vi "Create Token Request.vi"(4 "Code":string, 6 "State":string, 10 "Client":refnum<class "Client.lvclass">, 11 "Request in":refnum<class "Request.lvclass">) -> (1 "error out":errorcluster, 2 "POST Buffer":string, 3 "Request URL":string)   [LabVIEW 2020, in "OAuth2.lvlib" / "Request.lvclass"]
doc: "Internal VI for creating the URL and POST request body for performing a token request. This VI is only needed if implementing customized authorization flow functionality."
uses:
  Request.lvclass
  lv-http-util/HTTP Utils/HTTP Utils.lvlib
  Client/Client.lvclass
  lv-stream/stream/URI/URI.lvclass
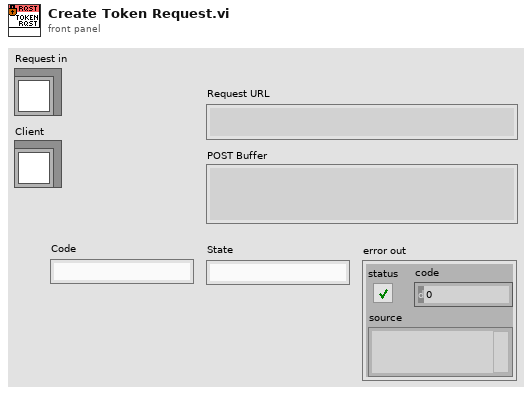
[diagram p1: front panel]
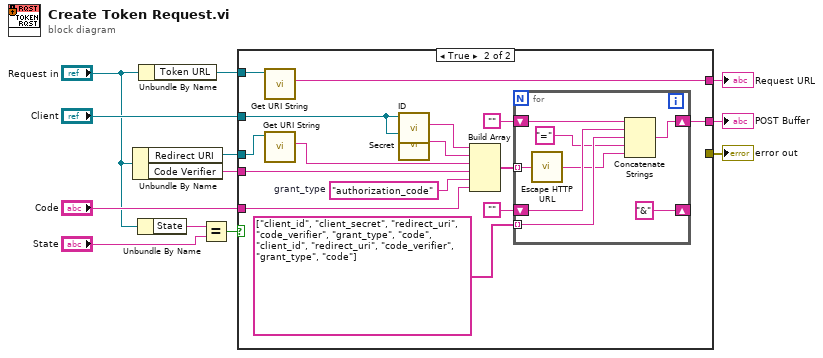
[diagram p0: block diagram]
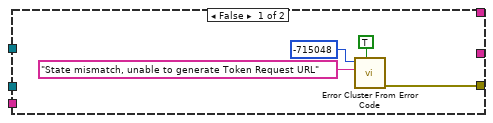
[diagram p2: hidden frame]
diagram:
  n1 = Unbundle By Name("Request in") -> ("Redirect URI"=w11:refnum<class "URI.lvclass">, "Code Verifier"=w8:string)
  n2 = Unbundle By Name("Request in") -> ("State"=w5:string)
  n3 = Unbundle By Name("Request in") -> ("Token URL"=w12:refnum<class "URI.lvclass">)
  n4 = Equal?(x=w5, y="State") -> (x = y?=w3:bool)
  n5 = case shown="True" w3 {
    tunnel: w12 -> [_ w20]
    tunnel: w11 -> [_ w22]
    tunnel: [_ w19] -> w10
    tunnel: "Client" -> [_ w27]
    tunnel: w8 -> [_ w26]
    tunnel: "Code" -> [_ w23]
    tunnel: [w14 _] -> w2
    tunnel: [_ w18] -> w1
    frame False {
      n6 = call <vilib>:"Error Cluster From Error Code.vi"("show call chain? (False)"=TRUE, "error message (\"\")"="State mismatch, unable to generate Token Request URL" ("error message (\"\")"), "error code (0)"=-715048) -> ("error out"=w14:errorcluster)  [unwired: 6 in]
    }
    frame True {
      w25 = "authorization_code"  # grant_type
      n7 = call "Get URI String.vi"("URI in"=w20) -> ("URI String"=w19:string)  [unwired: 8 in, 2 out]
      n8 = call "Get URI String.vi"("URI in"=w22) -> ("URI String"=w21:string)  [unwired: 8 in, 2 out]
      n9 = call "ID.vi"("Client in"=w27) -> ("Client ID"=w28:string)  [unwired: 10 in]
      n10 = call "Secret.vi"("Client in"=w27) -> ("Client Secret"=w17:string)  [unwired: 10 in]
      n11 = Build Array(w28, w17, w21, w26, w25, w23) -> (w31:string[])
      n12 = for {
        tunnel: w31 -> [w39] mode=indexing
        tunnel: string[] ["client_id", "client_secret", "redirect_uri", "code_verifier", "grant_type", "code", "client_id", "redirect_uri", "code_verifier", "grant_type", "code"] -> [w35] mode=indexing
        shift-right: ["&"] -> _
        shift-left: "" -> [w36]
        shift-right: [w32] -> w18
        shift-left: "" -> [w37]
        n13 = call "Escape HTTP URL.vi"("unescaped string in"=w39) -> ("escaped string out"=w33:string)
        n14 = Concatenate Strings(w37, w36, w35, "=" ("string"), w33) -> (w32:string)
      }
    }
  }
  "Request URL" <- w10
  "error out" <- w2
  "POST Buffer" <- w1
